vi "Winkel Lesen.vi"(8 "error IO":errorcluster, 10 "Task In":T2) -> (0 "error out":errorcluster, 2 "Winkel":T1)   [LabVIEW 2014]
uses:
  <vilib>/DAQmx/read.llb/DAQmx Read (Counter DBL 1Chan 1Samp).vi
  <vilib>/DAQmx/miscellaneous.llb/DAQmx Fill In Error Info.vi
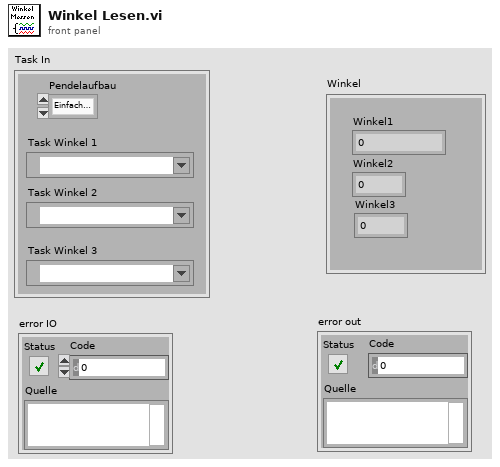
[diagram p1: front panel]
types:
  T1 = cluster{"Winkel1":dbl, "Winkel2":dbl, "Winkel3":dbl}
  T2 = cluster{"Pendelaufbau":enum16{"Einfachpendel", "Doppelpendel", "Dreifachpendel"}, "task/channels in":refnum<k21>, "task/channels in 2":refnum<k21>, "task/channels in 3":refnum<k21>}
  T3 = enum16{"Einfachpendel", "Doppelpendel", "Dreifachpendel"}
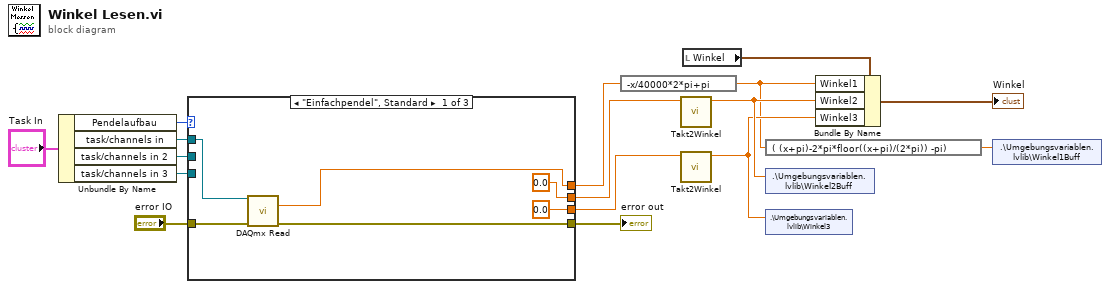
[diagram p0: block diagram]
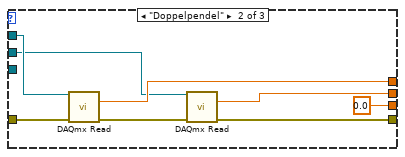
[diagram p2: hidden frame]
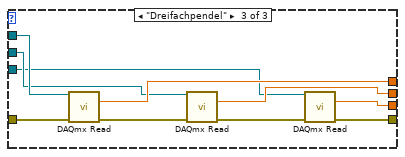
[diagram p3: hidden frame]
diagram:
  n1 = Unbundle By Name("Task In") -> ("Pendelaufbau"=w10:T3, "task/channels in"=w13:refnum<k21>, "task/channels in 2"=w12:refnum<k21>, "task/channels in 3"=w11:refnum<k21>)
  n2 = case shown="\"Einfachpendel\", Standard" w10 {
    tunnel: "error IO" -> [w22 w27 w39]
    tunnel: [w21 w29 w36] -> w15
    tunnel: w13 -> [w20 w26 w40]
    tunnel: [0.0 ("data") 0.0 ("data") w35] -> w7
    tunnel: [0.0 ("data") w24 w34] -> w5
    tunnel: [w19 w30 w33] -> w3
    tunnel: w12 -> [_ w25 w32]
    tunnel: w11 -> [_ _ w31]
    frame "Einfachpendel", Default {
      n3 = call-poly <vilib>:"DAQmx Read.vi"("task/channels in"=w20, "error in"=w22) -> ("data"=w19:dbl, "error out"=w21:errorcluster)  [unwired: 11 in, 1 out]
    }
    frame "Doppelpendel" {
      n4 = call-poly <vilib>:"DAQmx Read.vi"("task/channels in"=w26, "error in"=w27) -> ("data"=w30:dbl, "error out"=w28:errorcluster)  [unwired: 11 in, 1 out]
      n5 = call-poly <vilib>:"DAQmx Read.vi"("task/channels in"=w25, "error in"=w28) -> ("data"=w24:dbl, "error out"=w29:errorcluster)  [unwired: 11 in, 1 out]
    }
    frame "Dreifachpendel" {
      n6 = call-poly <vilib>:"DAQmx Read.vi"("task/channels in"=w40, "error in"=w39) -> ("data"=w33:dbl, "error out"=w38:errorcluster)  [unwired: 11 in, 1 out]
      n7 = call-poly <vilib>:"DAQmx Read.vi"("task/channels in"=w32, "error in"=w38) -> ("data"=w34:dbl, "error out"=w37:errorcluster)  [unwired: 11 in, 1 out]
      n8 = call-poly <vilib>:"DAQmx Read.vi"("task/channels in"=w31, "error in"=w37) -> ("data"=w35:dbl, "error out"=w36:errorcluster)  [unwired: 11 in, 1 out]
    }
  }
  "error out" <- w15
  n9 = expression code="-x/40000*2*pi+pi"(w3) -> (w1:dbl)
  n10 = call "Takt2Winkel.vi"("Taktzahl"=w5) -> ("Winkel (rad)"=w6:dbl)  [unwired: 10 in]
  n11 = call "Takt2Winkel.vi"("Taktzahl"=w7) -> ("Winkel (rad)"=w4:dbl)  [unwired: 10 in]
  n12 = local read "Winkel"() -> (w9:T1)
  n13 = expression code="( (x+pi)-2*pi*floor((x+pi)/(2*pi)) -pi)" ("Ausdrucksknoten")(w1) -> (w2:dbl)
  n14 = shared-variable ".\\Umgebungsvariablen.lvlib\\Winkel2Buff"(w6) -> ()  [unwired: 1 in, 1 out]
  n15 = shared-variable ".\\Umgebungsvariablen.lvlib\\Winkel3"(w4) -> ()  [unwired: 1 in, 1 out]
  n16 = Bundle By Name(cluster=w9, "Winkel1"=w1, "Winkel2"=w6, "Winkel3"=w4) -> (→"Winkel":T1)
  n17 = shared-variable ".\\Umgebungsvariablen.lvlib\\Winkel1Buff"(w2) -> ()  [unwired: 1 in, 1 out]
